vi "3d_Splint_Display.vi"() -> ()   [LabVIEW 2016]
panel:
  in  "stop":bool
  in  "User-Generated":dbl[](array[slide])=[35.84905660377358, 10.849056603773585, 12.264150943396226, 11.79245283018868] scale=0.0..100.0
  out "3D Picture":refnum<vi>(3d-picture)
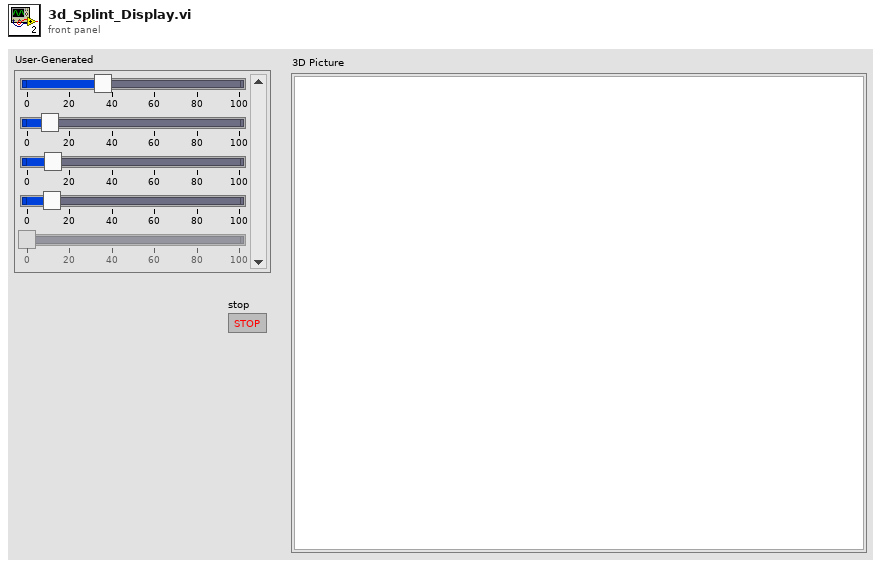
[diagram p1: front panel]
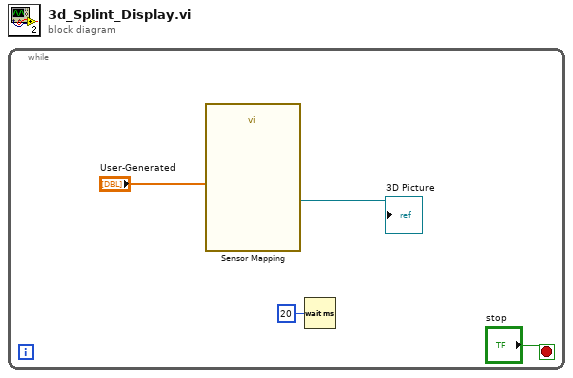
[diagram p0: block diagram]
diagram:
  n1 = while {
    stop <- "stop" stop-if-true
    n2 = call "Sensor Mapping"("Sensor Values"="User-Generated") -> ("Scene Ref Out"=→"3D Picture":refnum<vi>)  [unwired: 9 in, 1 out]
    n3 = Wait (ms)(milliseconds to wait=u32 20) -> ()  [unwired: 1 out]
  }
